vi "Set Inhibit.vi"(8 "error in (no error)":errorcluster, 10 "Inhibit (Off)":i32(ring) items=["Off", "Triggers", "AB", "AB and CD", "AB, CD and EF", "AB, CD, EF and GH"], 11 "VISA resource name":refnum<visa-resource-name>) -> (0 "error out":errorcluster, 3 "VISA resource name out":refnum<visa-resource-name>, 4 "Device Errors":cluster{"code":i32, "Text":string}[](array[cluster]))   [LabVIEW 2014, in "Stanford Research DG645 - Driver.lvlib"]
doc: "Trigger Command: INHB i\nInstrument Error Check\n\nSet the trigger inhibit state to i. The parameter i may be one of the following:\n\ni Inhibit\n0 Off\n1 Triggers\n2 AB\n3 AB and CD\n4 AB, CD and EF\n5 AB, CD, EF and GH\n\nThis command determines the behavior of the rear panal inhibit input. If the rear panel inhibit input is logic high when a trigger is detected, then the given channel dalays are inhibited."
uses:
  Stanford Research DG645 - Driver.lvlib
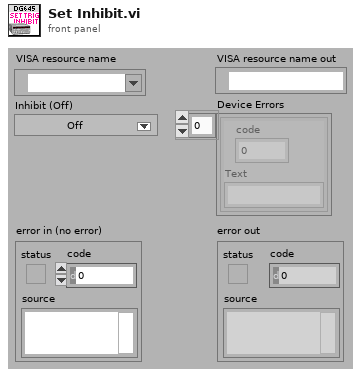
[diagram p1: front panel]
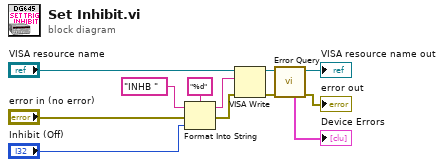
[diagram p0: block diagram]
diagram:
  n1 = Format Into String(format string="%d", initial string="INHB " ("command"), error in="error in (no error)", "Inhibit (Off)") -> (resulting string=w3:string, error out=w2:errorcluster)
  n2 = VISA Write(VISA resource name="VISA resource name", write buffer=w3, error in (no error)=w2) -> (VISA resource name out=w9:refnum<visa-resource-name>, error out=w6:errorcluster)  [unwired: 1 out]
  n3 = call "Error Query.vi"("error in (no error)"=w6, "VISA resource name"=w9) -> ("error out"=→"error out":errorcluster, "VISA resource name out"=→"VISA resource name out":refnum<visa-resource-name>, "Device Errors"=→"Device Errors":cluster{"code":i32, "Text":string}[])  [unwired: 7 in]
